vi "Gyro_wave_test.vi"() -> ()   [LabVIEW 2019]
uses:
  <vilib>/Analysis/3filter.llb/Filter Passband Type.ctl
  KNRm_ReMi_OS6_436Motor.lvlibp/BNO055_KNRm_ReMi.lvlib
  <vilib>/Analysis/NI_AALBase.lvlib
  <vilib>/ptbypt/NI_PtbyPt.lvlib
  KNRm_ReMi_OS6_436Motor.lvlibp
panel:
  in  "switch":bool
  in  "stop":bool
  out "Waveform Chart":dbl(graph)
  out "Filtered x":dbl format="%0.2f"
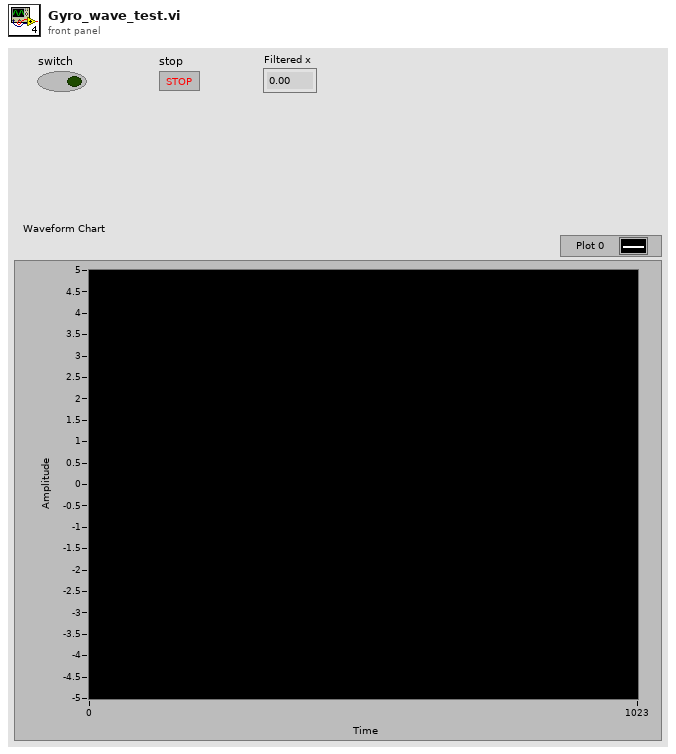
[diagram p1: front panel]
types:
  T1 = enum16{"ConfigMode", "ACC only", "Mag only", "Gyro only", "Acc Mag", "Acc Gyro", "Mag Gyro", "AMG", "Fusion IMU", "Fusion Compass", "Fusion M4G", "NDOF_FMC_OFF", "NDOF"}
  T2 = typedef "NI_AALBase.lvlib/Filter Passband Type.ctl" = enum32{"Lowpass", "Highpass", "Bandpass", "Bandstop"}
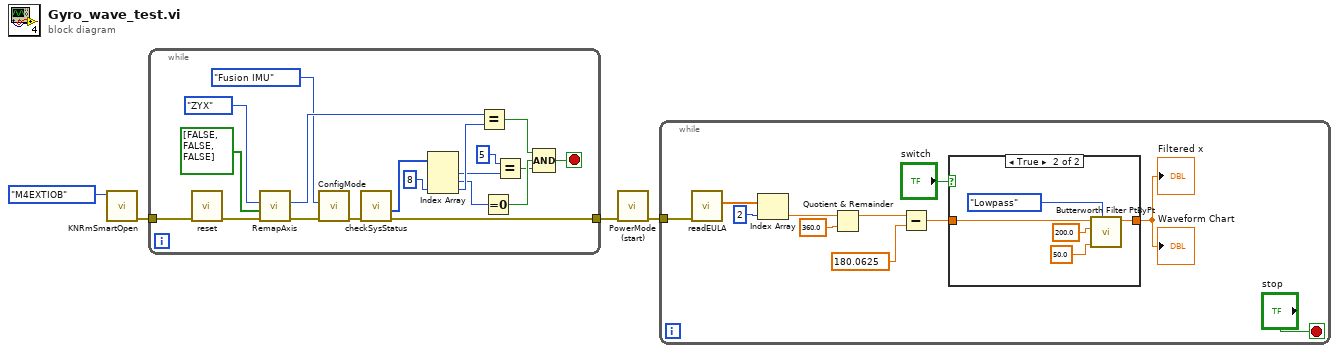
[diagram p0: block diagram]
diagram:
  n1 = call "KNRmSmartOpen.vi"("INI FPGA MODE"=enum16{"Original", "M4EXTIOB"}."M4EXTIOB") -> ("error out"=w4:errorcluster)  [unwired: 7 in, 3 out]
  n2 = while {
    tunnel: [w6] -> w2
    tunnel: w4 -> [w5]
    stop <- w22 stop-if-true
    n3 = call "reset.vi"("error in (no error)"=w5) -> ("error out"=w12:errorcluster)  [unwired: 10 in]
    n4 = call "RemapAxis.vi"("error in (no error)"=w12, "AxisSign [X, Y, Z] ( F:Pos, T:Neg)"=bool[] [FALSE, FALSE, FALSE], "AxisRemap [ Z, Y, X]"=enum16{"XYZ", "XZY", "YXZ", "YZX", "ZXY", "ZYX"}."ZYX" ("AxisRemap")) -> ("Error Out"=w9:errorcluster, "hexOut"=w11:u8)  [unwired: 7 in]
    n5 = call "ConfigMode.vi"("error in (no error)"=w9, "Mode"=T1."Fusion IMU") -> ("error out"=w8:errorcluster)  [unwired: 9 in]
    n6 = call "checkSysStatus.vi"("error in (no error)"=w8) -> ("error out"=w6:errorcluster, "System Status code"=w7:u8[])  [unwired: 8 in, 1 out]
    n7 = Index Array(array=w7, index #3=8 ("index")) -> (element #1=w19:u8, element #2=w17:u8, element #3=w20:u8)  [unwired: 2 in]
    n8 = Equal?(x=w11, y=w20) -> (x = y?=w23:bool)
    n9 = Equal To 0?(x=w17) -> (x = 0?=w16:bool)
    n10 = Equal?(x=u8 5, y=w19) -> (x = y?=w15:bool)
    n11 = Compound Arithmetic op=AND(w23, w16, w15) -> (w22:bool)
  }
  n12 = call "PowerMode (start).vi"("error in (no error)"=w2) -> ("error out"=w1:errorcluster)  [unwired: 10 in]
  n13 = while {
    tunnel: w1 -> [w24]
    stop <- "stop" stop-if-true
    n14 = call "readEULA.vi"("error in (no error)"=w24) -> ("EULA Output"=w32:dbl[])  [unwired: 9 in, 1 out]
    n15 = Index Array(array=w32, index=2) -> (element=w33:dbl)
    n16 = Quotient & Remainder(x=w33, y=360.0) -> (x-y*floor(x/y)=w30:dbl)  [unwired: 1 out]
    n17 = Subtract(x=w30, y=180.0625) -> (x-y=w29:dbl)
    n18 = case shown="True" "switch" {
      tunnel: w29 -> [w35 w40]
      tunnel: [w35 w39] -> w28
      frame False {
      }
      frame True {
        n19 = call <vilib>:"Butterworth Filter PtByPt.vi"("filter type"=Filter_Passband_Type."Lowpass", "low cutoff freq: fl"=50.0, "sampling freq: fs"=200.0, "x"=w40) -> ("Filtered x"=w39:dbl)  [unwired: 5 in, 1 out]
      }
    }
    "Filtered x" <- w28
    "Waveform Chart" <- w28
  }
